vi "Generate IOPub Events.vi"(8 "error in (no error)":errorcluster, 11 "object in":refnum<class "JuPyter_Client.lvclass">) -> (0 "error out":errorcluster, 3 "object out":refnum<class "JuPyter_Client.lvclass">)   [LabVIEW 2018, in "JuPyter_Client.lvclass"]
doc: "Designed to run as an asynch process, this will poll the IOPub socket until an error happens and generate Message Events"
uses:
  JuPyter_Client.lvclass
  <vilib>/addons/zeromq/poll_type.ctl
  Base Classes/Message Class/Message Class.lvclass
  <vilib>/addons/zeromq/zmq_poll_scalar.vi
  <vilib>/addons/zeromq/zmq_socket.lvclass
  <vilib>/addons/zeromq/zeromq.lvlib
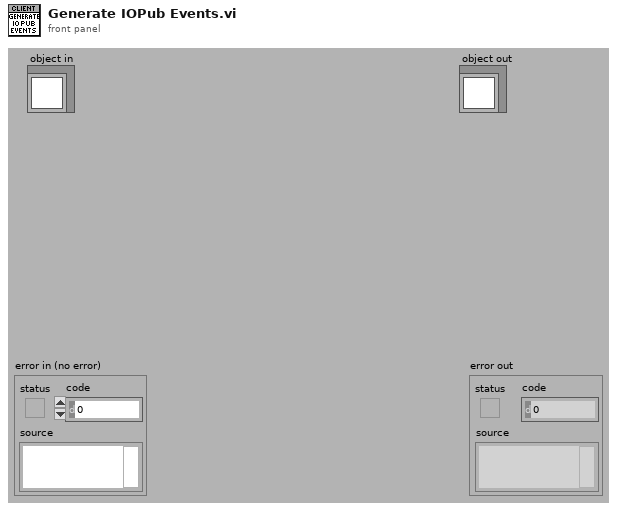
[diagram p1: front panel]
types:
  T1 = typedef "zeromq.lvlib/poll_type.ctl" = enum16{"None", "In", "Out", "In/Out"}
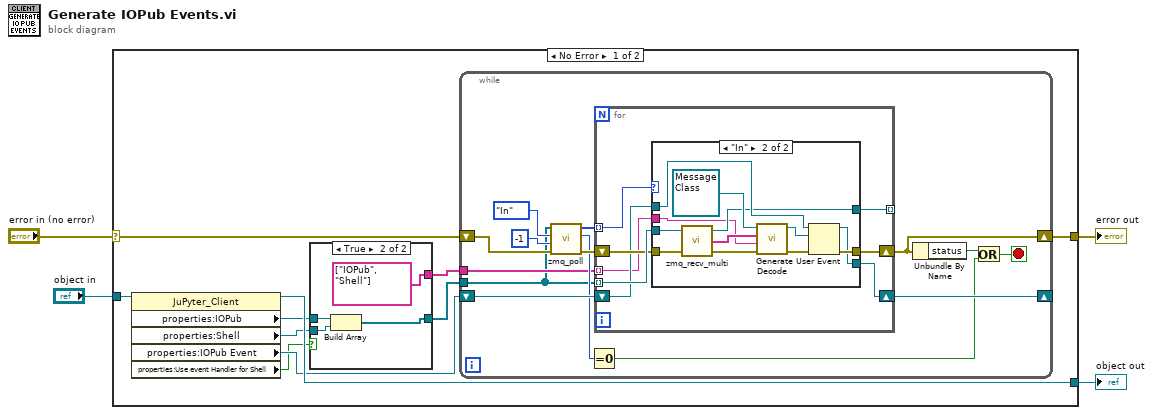
[diagram p0: block diagram]
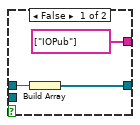
[diagram p2: hidden frame]
diagram:
  n1 = case shown="No Error" "error in (no error)" {
    selector: "error in (no error)" -> [w7 w60]
    tunnel: [w10 w60] -> w3
    tunnel: [w13 w59] -> w1
    tunnel: "object in" -> [w14 w59]
    frame No Error {
      n2 = property class="JuPyter_Client"(reference=w14) -> (reference out=w13:refnum<class "JuPyter_Client.lvclass">, "properties:IOPub"=w12:refnum<class "zmq_socket.lvclass">, "properties:Shell"=w8:refnum<class "zmq_socket.lvclass">, "properties:IOPub Event"=w11:refnum<user-event>, "properties:Use event Handler for Shell"=w9:bool)  [unwired: 1 in, 1 out]
      n3 = case shown="True" w9 {
        tunnel: [w16 w21] -> w6
        tunnel: w12 -> [w17 w20]
        tunnel: w8 -> [_ w19]
        tunnel: [string[] ["IOPub"] string[] ["IOPub", "Shell"]] -> w5
        frame False {
          n4 = Build Array(w17) -> (w16:refnum<class "zmq_socket.lvclass">[])
        }
        frame True {
          n5 = Build Array(w20, w19) -> (w21:refnum<class "zmq_socket.lvclass">[])
        }
      }
      n6 = while {
        shift-right: [w28] -> w10
        shift-left: w7 -> [w33]
        shift-right: [w30] -> _
        shift-left: w11 -> [w31]
        tunnel: w6 -> [w22]
        tunnel: w5 -> [w23]
        stop <- w25 stop-if-true
        n7 = call-poly <vilib>:"zmq_poll.vi"("error in"=w33, "timeout"=-1, "poll type"=poll_type."In", "sockets"=w22) -> ("error out"=w32:errorcluster, "nevents"=w29:i32, "polled events"=w34:T1[])  [unwired: 1 out]
        n8 = Equal To 0?(x=w29) -> (x = 0?=w26:bool)
        n9 = for {
          tunnel: w34 -> [w37] mode=indexing
          shift-right: [w40] -> w28
          shift-left: w32 -> [w42]
          shift-right: [w39] -> w30
          shift-left: w31 -> [w41]
          tunnel: w23 -> [w36] mode=indexing
          tunnel: w22 -> [w43] mode=indexing
          tunnel: [w38] -> _ mode=indexing
          n10 = case shown="\"In\"" w37 {
            tunnel: w43 -> [w45 w58]
            tunnel: w42 -> [w46 w57]
            tunnel: w41 -> [w44 w53]
            tunnel: [w46 w50] -> w40
            tunnel: [w44 w49] -> w39
            tunnel: [w45 w48] -> w38
            tunnel: w36 -> [_ w47]
            frame "None", Default {
            }
            frame "In" {
              n11 = call <vilib>:"zmq_recv_multi.vi"("error in"=w57, "socket in"=w58) -> ("error out"=w55:errorcluster, "parts"=w54:string[], "socket out"=w48:refnum<class "zmq_socket.lvclass">)  [unwired: 1 in]
              n12 = call "Decode.vi"("error in (no error)"=w55, "Socket"=w47, "Message In"=w54, "object in"=refnum<class "Message Class.lvclass"> refnum) -> ("error out"=w51:errorcluster, "object out"=w52:refnum<class "Message Class.lvclass">)  [unwired: 3 in, 3 out]
              n13 = Generate User Event(user event=w53, event data cluster=w52, error in=w51) -> (user event out=w49:refnum<user-event>, error out=w50:errorcluster)  [unwired: 1 in]
            }
          }
        }
        n14 = Unbundle By Name(w28) -> ("status"=w27:bool)
        n15 = Or(x=w27, y=w26) -> (x .or. y?=w25:bool)
      }
    }
    frame Error {
    }
  }
  "error out" <- w3
  "object out" <- w1
